vi "CIPeriodProps.vi"(5 "task in":refnum<k24>, 7 "error in (no error)":errorcluster) -> (0 "task out":refnum<k24>, 1 "StartingEdge":i32, 2 "Units":i32, 3 "error out":errorcluster, 4 "MeasurementTime":dbl)   [LabVIEW 2010]
uses:
  C:/Program Files/National Instruments/LabVIEW 2010/vi.lib/ULx/ULx_LV.dll
  Program Files/National Instruments/LabVIEW 2010/vi.lib/ULx/ULx_LV.dll
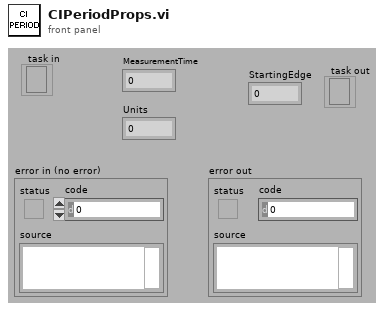
[diagram p1: front panel]
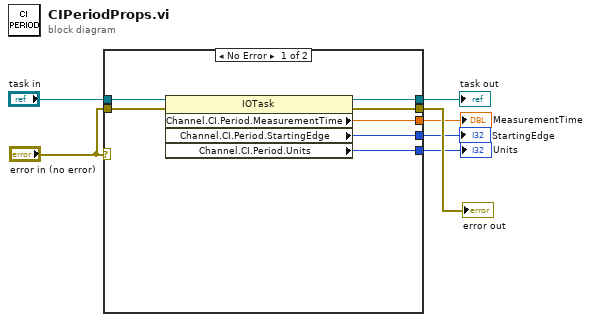
[diagram p0: block diagram]
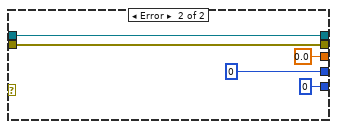
[diagram p2: hidden frame]
diagram:
  n1 = case shown="No Error" "error in (no error)" {
    tunnel: "task in" -> [w14 w19]
    tunnel: "error in (no error)" -> [w13 w18]
    tunnel: [w12 w19] -> w6
    tunnel: [w11 w18] -> w5
    tunnel: [w9 0 ("Channel.AI.Temp.Units")] -> w3
    tunnel: [w8 0 ("Channel.CI.Frequency.Units")] -> w1
    tunnel: [w10 0.0 ("Channel.CI.Frequency.MeasurementTime")] -> w2
    frame No Error {
      n2 = property class="IOTask"(reference=w14, error in=w13) -> (reference out=w12:refnum<k24>, error out=w11:errorcluster, "Channel.CI.Period.MeasurementTime"=w10:dbl, "Channel.CI.Period.StartingEdge"=w9:i32, "Channel.CI.Period.Units"=w8:i32)
    }
    frame Error {
    }
  }
  "task out" <- w6
  "error out" <- w5
  "StartingEdge" <- w3
  "MeasurementTime" <- w2
  "Units" <- w1
